vi "test Is OD Entry.vi"(11 "Test Case In":refnum<class "test Electronic Datasheet.lvclass">) -> (0 "error out":errorcluster, 3 "Test Case Out":refnum<class "test Electronic Datasheet.lvclass">)   [LabVIEW 2024, in "test Electronic Datasheet.lvclass"]
uses:
  test Electronic Datasheet.lvclass
  C:/Program Files/National Instruments/LabVIEW 2024/vi.lib/Astemes/LUnit/Test Case.lvclass
  <vilib>/Astemes/LUnit/Test Case.lvclass/Test Case.ctl
  e77553f5-9997-4175-9aac-2e0e77997e4c.vi
  <vilib>/Astemes/LUnit/Append Pass Result.vi
  <vilib>/Astemes/LUnit/Append Fail Result.vi
  <vilib>/Astemes/LUnit/Describe Comparison.vi
  e77553f5-9997-4175-9aac-2e0e77997e4c.vi/9c5d11cd-9439-4240-a1ee-d9baace9c924.vi
  <vilib>/Astemes/LUnit/Run In UI.vi
  <vilib>/Utility/error.llb/Clear Errors.vi
  <vilib>/Astemes/LUnit/Describe Variant.vi
  Core/Section Name/Section Name.lvclass
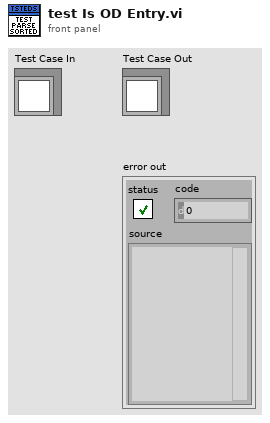
[diagram p1: front panel]
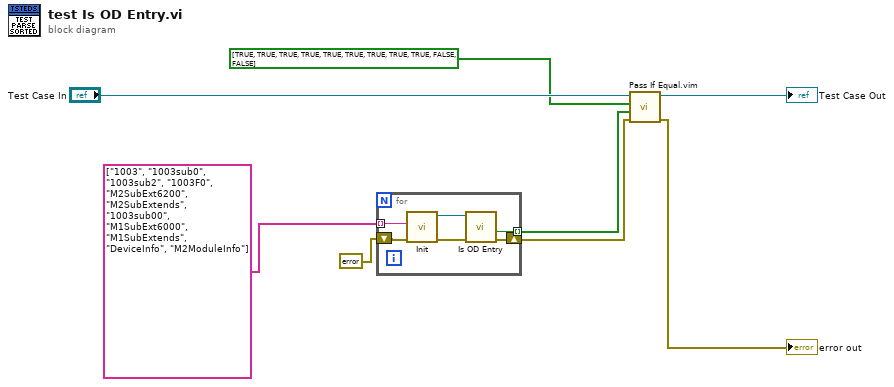
[diagram p0: block diagram]
diagram:
  n1 = for {
    tunnel: [w11] -> w2 mode=indexing
    tunnel: string[] ["1003", "1003sub0", "1003sub2", "1003F0", "M2SubExt6200", "M2SubExtends", "1003sub00", "M1SubExt6000", "M1SubExtends", "DeviceInfo", "M2ModuleInfo"] -> [w10] mode=indexing
    shift-right: [w12] -> w5
    shift-left: errorcluster {"status"=FALSE, "code"=0, "source"=""} ("error out") -> [w9]
    n2 = call "Init.vi"("error in"=w9, "Section Name"=w10) -> ("error out"=w13:errorcluster, "Section Name out"=w14:refnum<class "Section Name.lvclass">)  [unwired: 8 in]
    n3 = call "Is OD Entry.vi"("error in"=w13, "Section Name in"=w14) -> ("error out"=w12:errorcluster, "Is OD Entry?"=w11:bool)  [unwired: 5 in, 3 out]
  }
  n4 = call "Pass If Equal.vim"("error in (no error)"=w5, "Actual"=w2, "Expected"=bool[] [TRUE, TRUE, TRUE, TRUE, TRUE, TRUE, TRUE, TRUE, TRUE, FALSE, FALSE] ("Array"), "LUnit Test Case In"="Test Case In") -> ("error out"=→"error out":errorcluster, "LUnit Test Case Out"=→"Test Case Out":refnum<class "test Electronic Datasheet.lvclass">)  [unwired: 6 in]
